vi "sub_psk_demod.vi"(8 "index map":i32[](array[numeric]), 9 "symbol map":cdb[](array[numeric]), 11 "symbol":cdb[](array[numeric])) -> (3 "bitstream":i16[](array[numeric]))   [LabVIEW 2014]
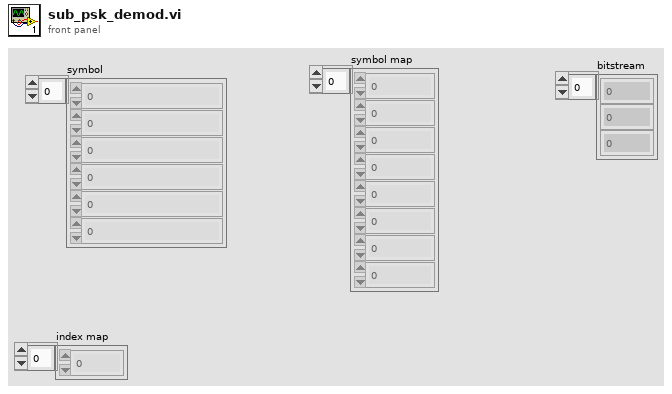
[diagram p1: front panel]
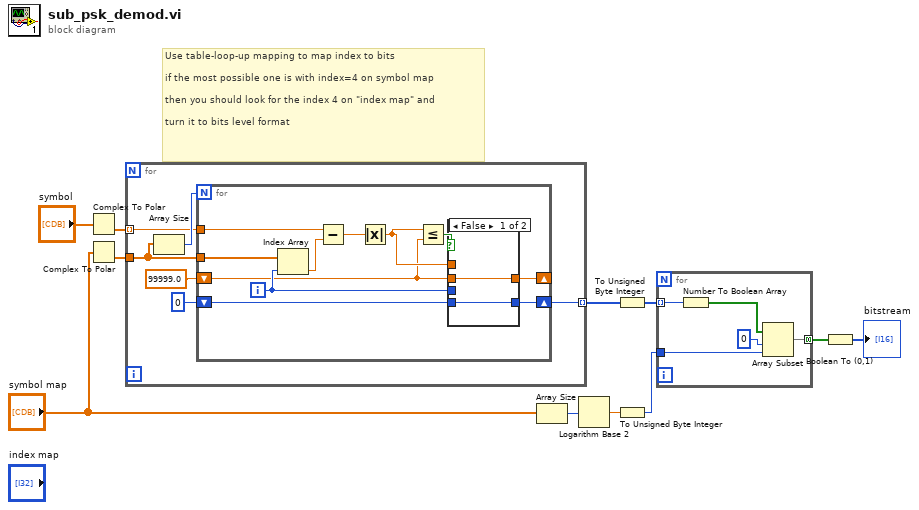
[diagram p0: block diagram]
diagram:
  # "Use table-loop-up mapping to map index to bits\n\nif the most possible one is with index=4 on symbol map\n\nthen you should look for the index 4 on \"index map\" and\n\nturn it to bits level format"
  n1 = Complex To Polar(r * e^(i*theta)="symbol") -> (theta=w10:dbl[])  [unwired: 1 out]
  n2 = Complex To Polar(r * e^(i*theta)="symbol map") -> (theta=w9:dbl[])  [unwired: 1 out]
  n3 = for {
    tunnel: w9 -> [w16]
    tunnel: w10 -> [w15] mode=indexing
    tunnel: [w12] -> w1 mode=indexing
    n4 = Array Size(array=w16) -> (size(s)=w17:i32)
    n5 = for {
      N: w17 -> [_]
      shift-right: [w24] -> _
      shift-left: 99999.0 -> [w19]
      tunnel: w16 -> [w28]
      tunnel: w15 -> [w27]
      shift-right: [w22] -> w12
      shift-left: 0 -> [w21]
      i -> [w23]
      n6 = Index Array(array=w28, index=w23) -> (element=w26:dbl)
      n7 = Subtract(x=w27, y=w26) -> (x-y=w25:dbl)
      n8 = Absolute Value(x=w25) -> (abs(x)=w20:dbl)
      n9 = Less Or Equal?(x=w20, y=w19) -> (x <= y?=w18:bool)
      n10 = case shown="False" w18 {
        tunnel: [w29 w32] -> w24
        tunnel: w20 -> [_ w32]
        tunnel: w23 -> [_ w31]
        tunnel: [w30 w31] -> w22
        tunnel: w19 -> [w29 _]
        tunnel: w21 -> [w30 _]
        frame False {
        }
        frame True {
        }
      }
    }
  }
  n11 = Array Size(array="symbol map") -> (size(s)=w8:i32)
  n12 = Logarithm Base 2(1:w8) -> (0:w7:dbl)
  n13 = To Unsigned Byte Integer(number=w1) -> (unsigned 8bit integer=w6:u8[])
  n14 = To Unsigned Byte Integer(number=w7) -> (unsigned 8bit integer=w5:u8)
  n15 = for {
    tunnel: w6 -> [w37] mode=indexing
    tunnel: w5 -> [w36]
    tunnel: [w34] -> w4 mode=concatenating
    n16 = Number To Boolean Array(number=w37) -> (Boolean array=w33:bool[])
    n17 = Array Subset(array=w33, index=0, length=w36) -> (w34:bool[])
  }
  n18 = Boolean To (0,1)(Boolean=w4) -> (0, 1=→"bitstream":i16[])
